vi "Data Channel.vi"(8 "error in (no error)":errorcluster, 11 "Node Ptr":T2 format="%.0x") -> (0 "error out":errorcluster)   [LabVIEW 2010, in "RefMem PtByPt Custom Device.lvlib"]
uses:
  RefMem PtByPt Custom Device.lvlib
  <vilib>/NI Veristand/Custom Device API/Custom Device Item Ref.ctl
  Controls/Data Channel Type.ctl
  <vilib>/NI Veristand/Custom Device API/Custom Device Channel Type.ctl
  Controls/Global.vi
  <vilib>/NI Veristand/Custom Device API/Get Item Property (U16).vi
  <vilib>/NI Veristand/Custom Device API/Get Item Property (U32).vi
  <vilib>/NI Veristand/Custom Device API/Set Item Property (U32).vi
  <vilib>/NI Veristand/Custom Device API/Set Item Property (U16).vi
  <vilib>/NI Veristand/Custom Device API/Custom Device API.lvlib
panel:
  in  "Default Value":dbl
  in  "Unit":string
  in  "Warning text":string="WARNING: The address selected by this channel is within the range of addresses reserved by NI VeriStand's built in reflective memory support!"
  out "Warn Icon":bool
  in  "Type":T1
  in  "Address":u32 format="%.0x"
  in  "Header":cluster{"Section Name":string}={"Section Name"="Data Channel"}
  in  "Description":string
  in  "Name":string
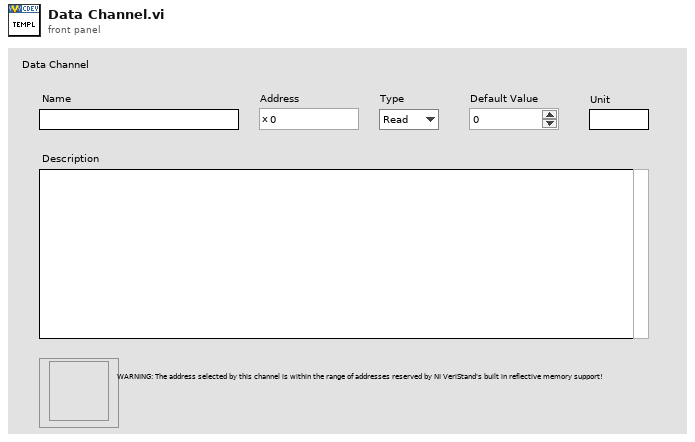
[diagram p1: front panel]
types:
  T1 = typedef "RefMem PtByPt Custom Device.lvlib/Data Channel Type.ctl" = enum16{"Read", "Write"}
  T2 = typedef "Custom Device API.lvlib/Custom Device Item Ref.ctl" = u64
  T3 = typedef "Custom Device API.lvlib/Custom Device Pointer.ctl" = refnum<k24>
  T4 = typedef "Custom Device API.lvlib/Custom Device Channel.ctl" = cluster{"Type":T5, "Units":string, "Default Value":dbl, "Faultable":bool, "Scalable":bool}
  T5 = typedef "Custom Device API.lvlib/Custom Device Channel Type.ctl" = enum16{"Input", "Output"}
  T6 = typedef "Custom Device API.lvlib/Custom Device Commands.ctl" = enum16{"Default", "Item renamed", "Shutdown", "Dynamic button pressed"}
  T7 = typedef "Custom Device API.lvlib/Custom Device Item Info.ctl" = cluster{"Name":string, "Is Channel":bool, "GUID":string}
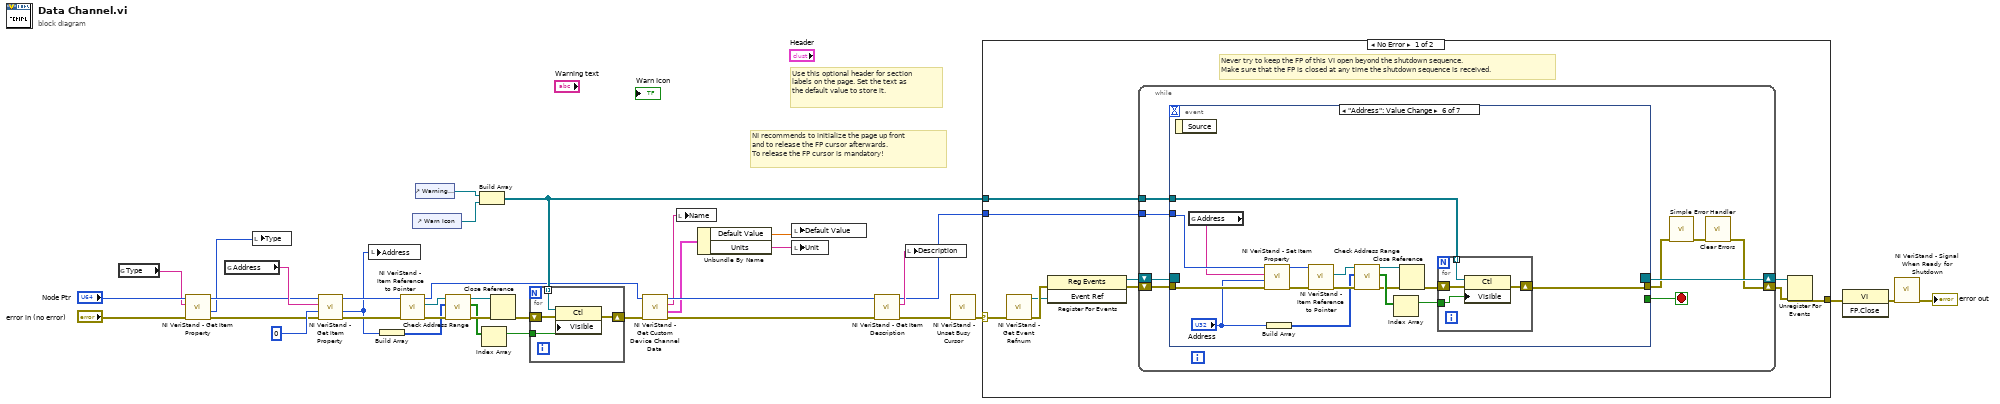
[diagram p0: block diagram]
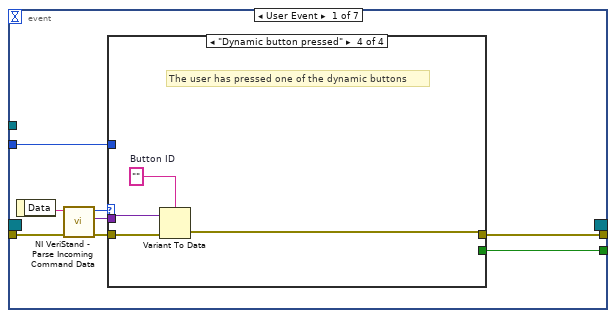
[diagram p2: hidden frame]
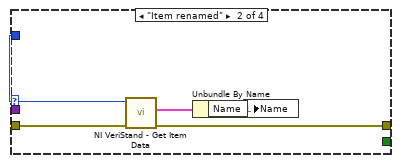
[diagram p4: hidden frame]
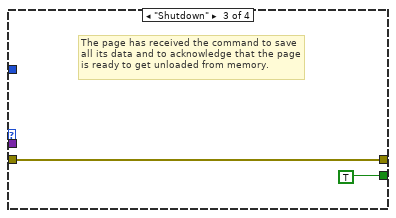
[diagram p5: hidden frame]
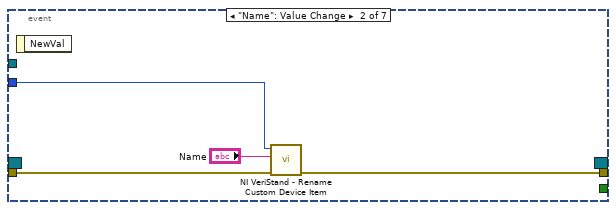
[diagram p6: hidden frame]
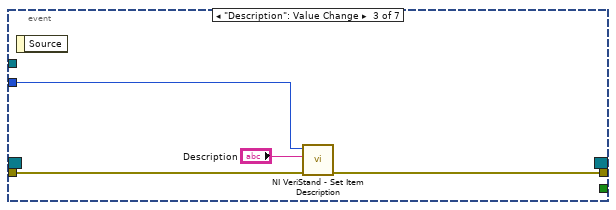
[diagram p7: hidden frame]
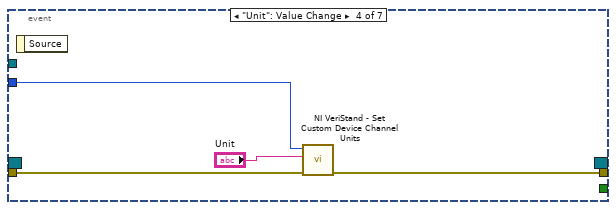
[diagram p8: hidden frame]
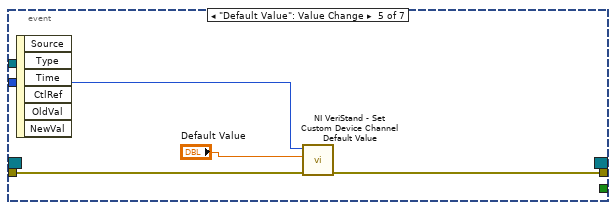
[diagram p9: hidden frame]
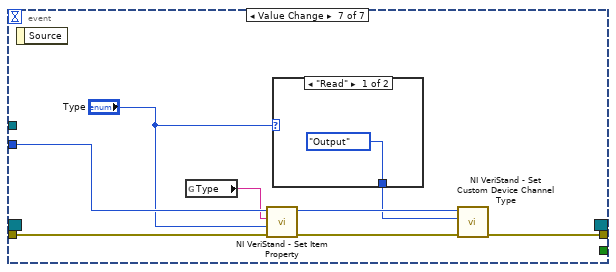
[diagram p10: hidden frame]
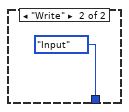
[diagram p11: hidden frame]
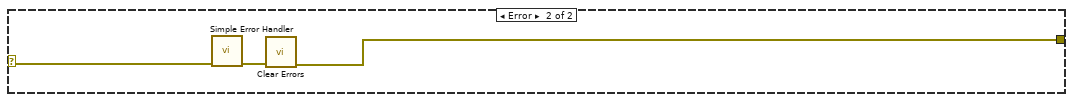
[diagram p12: hidden frame]
diagram:
  # "Use this optional header for section labels on the page. Set the text as the default value to store it."
  # "NI recommends to initialize the page up front\nand to release the FP cursor afterwards.\nTo release the FP cursor is mandatory!"
  n1 = global read "Global.vi" "Type"() -> (w14:string)
  n2 = call-poly <vilib>:"NI VeriStand - Get Item Property.vi"("error in (no error)"="error in (no error)", "Property Name"=w14, "Item Ref in"="Node Ptr") -> ("error out"=w16:errorcluster, "Value"=w13:u16, "Item Ref out"=w15:T2)  [unwired: 5 in, 1 out]
  n3 = global read "Global.vi" "Address"() -> (w32:string)
  n4 = local write "Type"(w13) -> ()
  n5 = call-poly <vilib>:"NI VeriStand - Get Item Property.vi"("error in (no error)"=w16, "Default Value"=u32 0 ("Address"), "Property Name"=w32, "Item Ref in"=w15) -> ("error out"=w30:errorcluster, "Value"=w26:u32, "Item Ref out"=w29:T2)  [unwired: 4 in, 1 out]
  n6 = local write "Address"(w26) -> ()
  n7 = Build Array(w26) -> (w2:u32[])
  n8 = call <vilib>:"NI VeriStand - Item Reference to Pointer.vi"("error in (no error)"=w30, "Item Ref in"=w29) -> ("error out"=w28:errorcluster, "Node Pointer"=w27:T3, "Item Ref out"=w11:T2)  [unwired: 6 in, 1 out]
  n9 = control-ref of="Warn Icon"() -> (w22:refnum<vi>)
  n10 = control-ref of="Warning text"() -> (w21:refnum<vi>)
  n11 = call "Check Address Range.vi"("error in (no error)"=w28, "Addresses"=w2, "Node Pointer In"=w27) -> ("error out"=w25:errorcluster, "Inside NIVS Range"=w20:bool[], "Node Pointer dup"=w24:T3)  [unwired: 6 in]
  n12 = Build Array(w21, w22) -> (w19:refnum<vi>[])
  n13 = Index Array(array=w20) -> (element=w1:bool)  [unwired: 1 in]
  n14 = Close Reference(reference=w24, error in (no error)=w25) -> (error out=w23:errorcluster)
  n15 = for {
    shift-right: [w38] -> w12
    shift-left: w23 -> [w41]
    tunnel: w19 -> [w40] mode=indexing
    tunnel: w1 -> [w39]
    n16 = property on="Property Node" class="Ctl"(reference=w40, error in=w41, "Visible"=w39) -> (error out=w38:errorcluster)  [unwired: 1 out]
  }
  n17 = call <vilib>:"NI VeriStand - Get Custom Device Channel Data.vi"("error in (no error)"=w12, "Channel Ref in"=w11) -> ("error out"=w10:errorcluster, "Channel"=w8:T4, "Channel Name"=w5:string, "Channel Ref out"=w9:T2)  [unwired: 4 in, 2 out]
  n18 = local write "Name"(w5) -> ()
  n19 = Unbundle By Name(w8) -> ("Default Value"=w3:dbl, "Units"=w4:string)
  n20 = local write "Default Value"(w3) -> ()
  n21 = local write "Unit"(w4) -> ()
  n22 = call <vilib>:"NI VeriStand - Get Item Description.vi"("error in (no error)"=w10, "Item Ref in"=w9) -> ("error out"=w7:errorcluster, "Description"=w33:string, "Item Ref out"=w6:T2)  [unwired: 7 out]
  n23 = local write "Description"(w33) -> ()
  n24 = call <vilib>:"NI VeriStand - Unset Busy Cursor.vi"("error in (no error)"=w7) -> ("error out"=w34:errorcluster)  [unwired: 10 out]
  n25 = case shown="No Error" w34 {
    selector: w34 -> [w43 w129]
    tunnel: [w48 w127] -> w37
    tunnel: w6 -> [w44 _]
    tunnel: w19 -> [w42 _]
    frame No Error {
      # "Never try to keep the FP of this VI open beyond the shutdown sequence.\nMake sure that the FP is closed at any time the shutdown sequence is received."
      n26 = call <vilib>:"NI VeriStand - Get Event Refnum.vi"("error in (no error)"=w43) -> ("error out"=w51:errorcluster, "Event Ref"=w47:refnum<user-event>)  [unwired: 9 out]
      n27 = register-events(error in=w51, w47) -> (reference out=w45:refnum<event-registration>, error out=w46:errorcluster)  [unwired: 1 in]
      n28 = while {
        tunnel: w44 -> [w56]
        shift-right: [w53] -> w49
        shift-left: w46 -> [w59]
        shift-right: [w60] -> w50
        shift-left: w45 -> [w58]
        tunnel: w42 -> [w52]
        stop <- w57 stop-if-true
        n29 = event shown="[5] \"Address\": Value Change" {
          selector: w58 -> [_ _ _ _ _ _ _]
          dyn-events: [_ _ _ _ _ _ _] -> w60
          timeout: _ -> [_ _ _ _ _ _ _]
          tunnel: w59 -> [w68 w84 w87 w91 w95 w112 w124]
          tunnel: [w64 _ _ _ _ _ _] -> w57
          tunnel: [w63 w83 w86 w90 w94 w99 w119] -> w55
          tunnel: w56 -> [w62 w82 w88 w92 w96 w111 w123]
          tunnel: w52 -> [_ _ _ _ _ w100 _]
          event User Event {
            n30 = event-data() -> ("Data"=w67:string)  [unwired: 1 out]
            n31 = call <vilib>:"NI VeriStand - Parse Incoming Command Data.vi"("error in (no error)"=w68, "Data"=w67) -> ("error out"=w66:errorcluster, "Data"=w61:variant, "Action"=w65:T6)  [unwired: 7 out]
            n32 = case shown="\"Dynamic button pressed\"" w65 {
              tunnel: w66 -> [w69 w74 w75 w80]
              tunnel: [_ _ TRUE _] -> w64
              tunnel: [w69 w71 w75 w77] -> w63
              tunnel: w62 -> [_ w73 _ _]
              tunnel: w61 -> [_ _ _ w79]
              frame "Default", Default {
              }
              frame "Item renamed" {
                n33 = call <vilib>:"NI VeriStand - Get Item Data.vi"("error in (no error)"=w74, "Item Ref in"=w73) -> ("error out"=w71:errorcluster, "Item Info"=w72:T7)  [unwired: 8 out]
                n34 = Unbundle By Name(w72) -> ("Name"=w70:string)
                n35 = local write "Name"(w70) -> ()
              }
              frame "Shutdown" {
                # "The page has received the command to save all its data and to acknowledge that the page is ready to get unloaded from memory."
              }
              frame "Dynamic button pressed" {
                w78 = ""  # Button ID
                # "The user has pressed one of the dynamic buttons"
                n36 = Variant To Data(error in=w80, Variant=w79, type=w78) -> (error out=w77:errorcluster)  [unwired: 1 out]
              }
            }
          }
          event "Name": Value Change {
            n37 = event-data() -> ()  [unwired: 2 out]
            n38 = call <vilib>:"NI VeriStand - Rename Custom Device Item.vi"("error in (no error)"=w84, "New Name"="Name", "Item Ref in"=w82) -> ("error out"=w83:errorcluster)  [unwired: 8 out]
          }
          event "Description": Value Change {
            n39 = event-data() -> ()  [unwired: 2 out]
            n40 = call <vilib>:"NI VeriStand - Set Item Description.vi"("error in (no error)"=w87, "Description"="Description", "Item Ref in"=w88) -> ("error out"=w86:errorcluster)  [unwired: 8 out]
          }
          event "Unit": Value Change {
            n41 = event-data() -> ()  [unwired: 2 out]
            n42 = call <vilib>:"NI VeriStand - Set Custom Device Channel Units.vi"("error in (no error)"=w91, "Units"="Unit", "Channel Ref in"=w92) -> ("error out"=w90:errorcluster)  [unwired: 7 in, 1 out]
          }
          event "Default Value": Value Change {
            n43 = event-data() -> ()  [unwired: 7 out]
            n44 = call <vilib>:"NI VeriStand - Set Custom Device Channel Default Value.vi"("error in (no error)"=w95, "Default Value"="Default Value", "Channel Ref in"=w96) -> ("error out"=w94:errorcluster)  [unwired: 7 in, 1 out]
          }
          event "Address": Value Change {
            n45 = event-data() -> ()  [unwired: 2 out]
            n46 = global read "Global.vi" "Address"() -> (w110:string)
            n47 = call-poly <vilib>:"NI VeriStand - Set Item Property.vi"("error in (no error)"=w112, "Value"="Address", "Property Name"=w110, "Item Ref in"=w111) -> ("error out"=w102:errorcluster, "Item Ref out"=w101:T2)  [unwired: 5 in, 1 out]
            n48 = Build Array("Address") -> (w98:u32[])
            n49 = call <vilib>:"NI VeriStand - Item Reference to Pointer.vi"("error in (no error)"=w102, "Item Ref in"=w101) -> ("error out"=w104:errorcluster, "Node Pointer"=w105:T3)  [unwired: 6 in, 2 out]
            n50 = call "Check Address Range.vi"("error in (no error)"=w104, "Addresses"=w98, "Node Pointer In"=w105) -> ("error out"=w106:errorcluster, "Inside NIVS Range"=w109:bool[], "Node Pointer dup"=w107:T3)  [unwired: 6 in]
            n51 = Index Array(array=w109) -> (element=w97:bool)  [unwired: 1 in]
            n52 = Close Reference(reference=w107, error in (no error)=w106) -> (error out=w108:errorcluster)
            n53 = for {
              shift-right: [w113] -> w99
              shift-left: w108 -> [w116]
              tunnel: w100 -> [w115] mode=indexing
              tunnel: w97 -> [w114]
              n54 = property on="Property Node" class="Ctl"(reference=w115, error in=w116, "Visible"=w114) -> (error out=w113:errorcluster)  [unwired: 1 out]
            }
          }
          event Value Change {
            n55 = event-data() -> ()  [unwired: 2 out]
            n56 = global read "Global.vi" "Type"() -> (w122:string)
            n57 = call-poly <vilib>:"NI VeriStand - Set Item Property.vi"("error in (no error)"=w124, "Value"="Type", "Property Name"=w122, "Item Ref in"=w123) -> ("error out"=w121:errorcluster, "Item Ref out"=w120:T2)  [unwired: 5 in, 1 out]
            n58 = case shown="\"Read\"" "Type" {
              tunnel: [Custom_Device_Channel_Type."Output" ("Type") Custom_Device_Channel_Type."Input" ("Type")] -> w117
              frame "Read" {
              }
              frame "Write" {
              }
            }
            n59 = call <vilib>:"NI VeriStand - Set Custom Device Channel Type.vi"("error in (no error)"=w121, "Type"=w117, "Channel Ref in"=w120) -> ("error out"=w119:errorcluster)  [unwired: 7 in, 1 out]
          }
        }
        n60 = call <vilib>:"Simple Error Handler.vi"("error in (no error)"=w55) -> ("error out"=w54:errorcluster)  [unwired: 1 in, 7 out]
        n61 = call <vilib>:"Clear Errors.vi"("error in (no error)"=w54) -> ("error out"=w53:errorcluster)  [unwired: 6 out]
      }
      n62 = Unregister For Events(event registration refnum=w50, error in=w49) -> (error out=w48:errorcluster)
    }
    frame Error {
      n63 = call <vilib>:"Simple Error Handler.vi"("error in (no error)"=w129) -> ("error out"=w128:errorcluster)  [unwired: 1 in, 7 out]
      n64 = call <vilib>:"Clear Errors.vi"("error in (no error)"=w128) -> ("error out"=w127:errorcluster)  [unwired: 6 out]
    }
  }
  n65 = invoke class="VI" method="FP.Close"(error in=w37) -> (error out=w36:errorcluster)  [unwired: 2 in, 2 out]
  n66 = call <vilib>:"NI VeriStand - Signal When Ready for Shutdown.vi"("error in (no error)"=w36) -> ("error out"=→"error out":errorcluster)  [unwired: 10 out]
